vi "ST_parse_ST50_results_response.vi"(6 "recordset_in":variant[][](array[variant]), 7 "Part exists?":bool, 8 "error_in":errorcluster, 11 "command_nmb":u8) -> (0 "error_out":errorcluster, 3 "reference_data_to_PLC":u8[](array[numeric]))   [LabVIEW 2020]
uses:
  _misc/byte_array_parser/from_SGL.vi
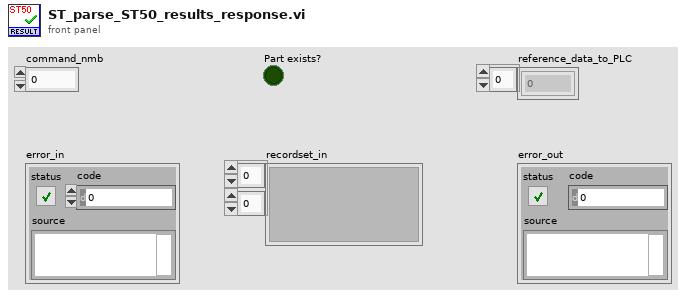
[diagram p1: front panel]
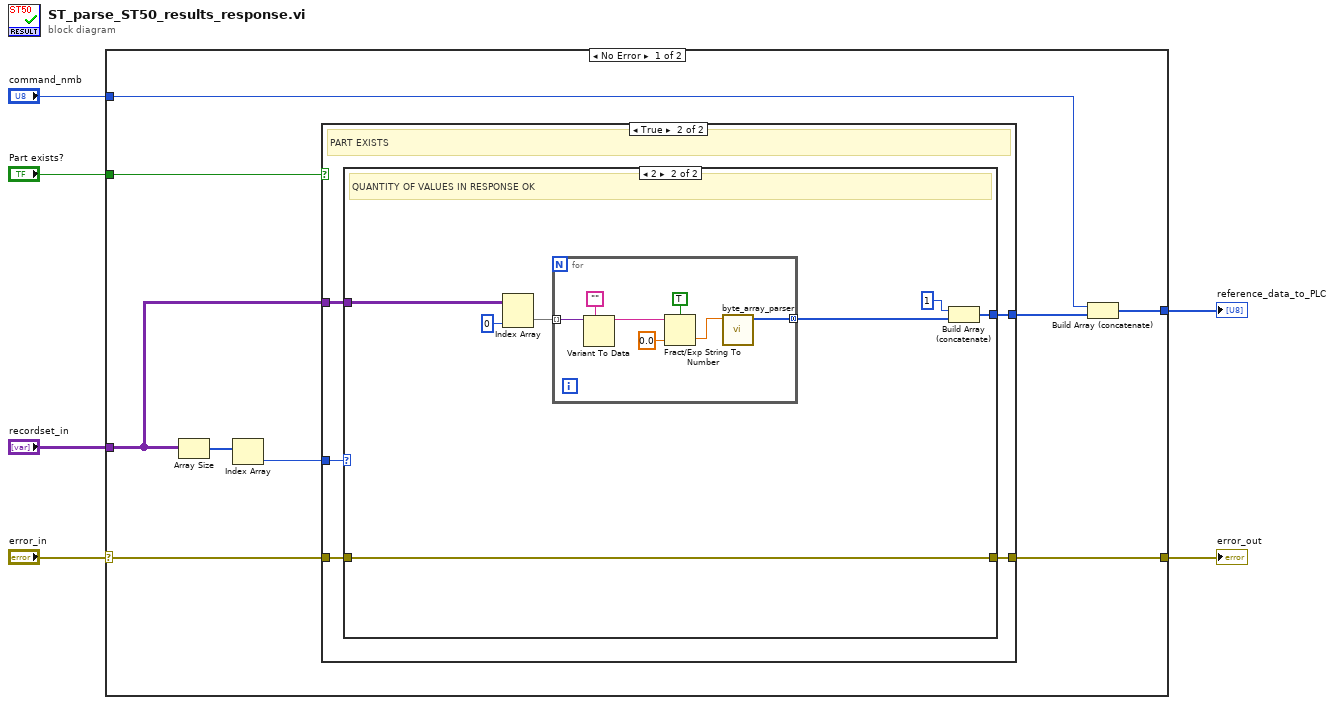
[diagram p0: block diagram]
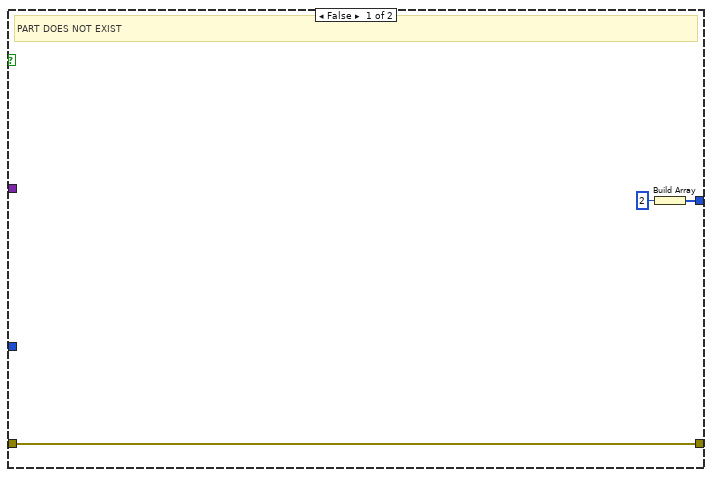
[diagram p2: hidden frame]
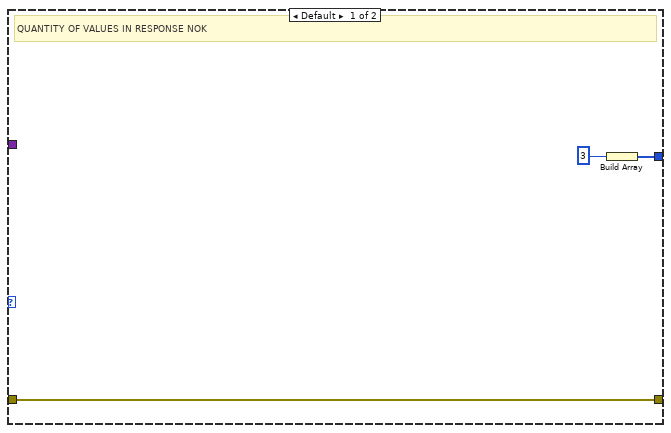
[diagram p3: hidden frame]
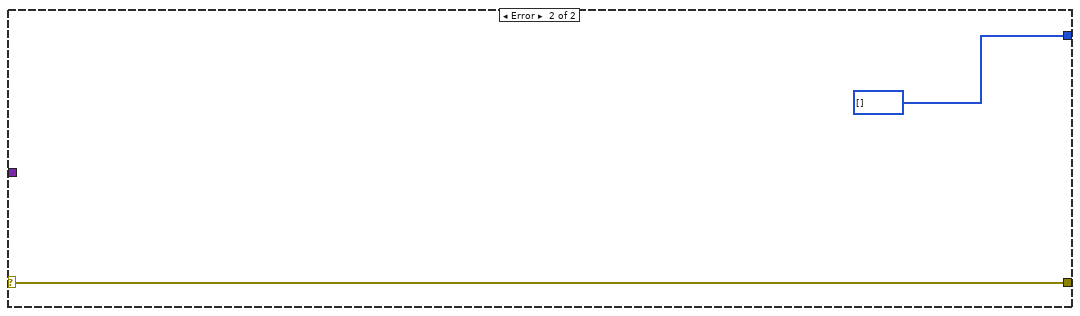
[diagram p4: hidden frame]
diagram:
  n1 = case shown="No Error" "error_in" {
    selector: "error_in" -> [w13 w42]
    tunnel: [w15 u8[] []] -> w2
    tunnel: "command_nmb" -> [w14 _]
    tunnel: "recordset_in" -> [w7 _]
    tunnel: [w12 w42] -> w3
    tunnel: "Part exists?" -> [w10 _]
    frame No Error {
      n2 = Array Size(array=w7) -> (size(s)=w9:i32[])
      n3 = Index Array(array=w9) -> (element=w8:i32)  [unwired: 1 in]
      n4 = case shown="True" w10 {
        tunnel: [w16 w23] -> w11
        tunnel: w13 -> [w18 w22]
        tunnel: [w18 w21] -> w12
        tunnel: w8 -> [_ w20]
        tunnel: w7 -> [_ w19]
        frame False {
          # "PART DOES NOT EXIST"
          n5 = Build Array(u8 2) -> (w16:u8[])
        }
        frame True {
          # "PART EXISTS"
          n6 = case shown="2" w20 {
            tunnel: [w24 w31] -> w23
            tunnel: w22 -> [w26 w33]
            tunnel: [w26 w33] -> w21
            tunnel: w19 -> [_ w27]
            frame Default {
              # "QUANTITY OF VALUES IN RESPONSE NOK"
              n7 = Build Array(u8 3) -> (w24:u8[])
            }
            frame 2 {
              # "QUANTITY OF VALUES IN RESPONSE OK"
              n8 = Index Array(array=w27, index (col)=0 ("index (row)")) -> (element=w30:variant[])  [unwired: 1 in]
              n9 = for {
                tunnel: w30 -> [w35] mode=indexing
                tunnel: [w37] -> w29 mode=concatenating
                n10 = Variant To Data(type="", Variant=w35) -> (data=w34:string)  [unwired: 1 in, 1 out]
                n11 = Fract/Exp String To Number(use system decimal point (T)=TRUE, string=w34, default (0 dbl)=sgl 0.0 ("index")) -> (number=w39:sgl)  [unwired: 1 in, 1 out]
                n12 = call-poly "byte_array_parser.vi"("I16"=w39) -> ("byte_array"=w37:u8[])  [unwired: 9 in, 1 out]
              }
              n13 = Build Array (concatenate)(u8 1, w29) -> (w31:u8[])
            }
          }
        }
      }
      n14 = Build Array (concatenate)(w14, w11) -> (w15:u8[])
    }
    frame Error {
    }
  }
  "error_out" <- w3
  "reference_data_to_PLC" <- w2
